vi "Module_p_control_v1.vi"() -> ()   [LabVIEW 2014]
uses:
  <vilib>/rvi/FXPMathLib/FxpSinAndCos/XNode/nifxpmath_SinAndCos.xnode
  <vilib>/eio/EIONode/EIONode.xnode
  <vilib>/rvi/FXPMathLib/FxpMul/XNode/nifxpmath_Multiplier.xnode
  <vilib>/rvi/FXPMathLib/FxpSinAndCos/simVIs/DllFxpSinAndCosTemp_sub.vi
  <vilib>/rvi/FXPMathLib/FxpSinAndCos/subVIs/nifxpmath_SinAndCos_SimConfig.ctl
  <vilib>/rvi/eio/common/nirviEmuTemplateMethod_errors.vi
  <vilib>/rvi/FXPMathLib/sim/FxpSim.dll
  <vilib>/rvi/DataTransferAndStorage/Container/XNode/niFpgaContainer.xnode
  <vilib>/rvi/FXPMathLib/FxpSub/XNode/nifxpmath_Sub.xnode
  <vilib>/rvi/FXPMathLib/FxpAdd/XNode/nifxpmath_Add.xnode
  <vilib>/rvi/Analysis/measure/butterworth/XNode/niFpgaButterworthFilter.xnode
  <vilib>/rvi/FXPMathLib/FxpAtan2/XNode/nifxpmath_Atan2.xnode
  <vilib>/rvi/FXPMathLib/FxpAtan2/simVIs/DllFxpAtan2Temp_sub.vi
  <vilib>/rvi/FXPMathLib/FxpAtan2/subVIs/nifxpmath_Atan2_SimConfig.ctl
  <vilib>/rvi/interface/RandomDataEmulation/nirviRandomDataFpgaMultiElementTemplate.vi
panel:
  out "Omega_p(M_avg)":fxp<+/-,57,22>
  out "Omega_p(M)":fxp<+/-,32,18>
  out "rad(NrTheta)_p":fxp<+/-,33,18>
  out "Encoder_Position_p":i32
  in  "fb_limit":fxp<+,16,11>
  in  "Dy_d_M_avg_Tc (uSec)":u32 caption="M_avg_Tc (uSec)"
  in  "Method case 2":i32
  out "Omega_b(rad/s)":fxp<+/-,32,18>
  out "Omega_y(M_avg)":fxp<+/-,32,18>
  out "Omega_y(M)":fxp<+/-,32,18>
  in  "Count(s)":u32
  out "Boolean":bool
  out "Db_temp":fxp<+/-,22,7>
  in  "Sin ini":bool
  out "xb_dd":fxp<+/-,25,15>
  in  "scaled coefficients_xb_dd":i32[](array[numeric])=[1067016412, 3362706]
  out "Db_dd":fxp<+/-,25,15>
  in  "scaled coefficients_Db_dd":i32[](array[numeric])=[1067016412, 3362706]
  out "Dab_edd":fxp<+/-,34,12>
  out "Dab_ed":fxp<+/-,33,10>
  out "fbr":fxp<+/-,20,10>
  in  "Kvb":fxp<+,15,8>
  in  "Bvb":fxp<+,15,8>
  out "Dab_e":fxp<+/-,26,11>
  in  "Dbr":fxp<+/-,22,8>
  in  "Inv./Pos.":bool
  out "Dabr_sin/cos":fxp<+/-,22,8>
  in  "Sin_offset_b":fxp<+/-,12,8>
  in  "Sin_magnitude_b":fxp<+/-,11,8>
  out "Dabr_d":fxp<+/-,33,10>
  out "Sin_omega":fxp<+,29,9>
  out "Dabr_dd":fxp<+/-,34,12>
  in  "Sin wave frenqueny (Hz)":fxp<+,21,5>
  out "Dy_d(M_avg method)":fxp<+/-,32,12>
  in  "Dy_d_M_Tc (mSec)":u32 format="%#_6f"
  out "Dy_d(M method)":fxp<+/-,32,12>
  out "Dp_d(M_avg method)":fxp<+/-,25,10>
  in  "Dp_d_M_avg_Tc (uSec)":u32 caption="M_avg_Tc (uSec)"
  out "Dp_d(M method)":fxp<+/-,25,10>
  in  "Dp_d_M_Tc (mSec)":u32 format="%#_6f"
  in  "Method case":i32
  out "xb_d(T method)":fxp<+/-,25,10>
  out "Dy_d(T method)":fxp<+/-,32,12>
  in  "mt0_velocity":u32
  out "mt_velocity":u32
  in  "mt0_omega":u32
  out "mt_omega":u32
  out "fbt_d":fxp<+/-,25,15>
  out "Db_d(mm/s)":fxp<+/-,32,12>
  out "xb_d(mm/s)":fxp<+/-,25,10>
  in  "dFb_PID_add":bool
  in  "scaled coefficients_dFb_PID":i32[](array[numeric])=[1067016412, 3362706]
  out "dFb_PID":fxp<+/-,25,15>
  out "Sin wave time (s)":fxp<+,64,32>
  in  "Encoder Reset_p":bool
  out "Dp(mm)":fxp<+/-,22,7>
  in  "Friction tolerance_b":fxp<+,12,4>
  in  "Coe Ini":bool
  in  "Encoder Reset_y":bool
  in  "Stop Motor_b":bool
  in  "viscous_cons_b":fxp<+/-,20,10>
  in  "fstb":fxp<+/-,15,6>
  in  "Db_d_tol":fxp<+,20,12>
  in  "Kib":fxp<+,27,10>
  in  "Kdb":fxp<+,26,2>
  in  "kb c":fxp<+,15,8>
  in  "kb t":fxp<+,15,8>
  out "fbt_i":fxp<+/-,34,18>
  in  "Kpb":fxp<+,11,7>=0.375
  in  "fv_coeff. b":fxp<+,13,1>
  out "Friction comp_b":fxp<+/-,20,10>
  in  "fcb":fxp<+/-,15,6>
  in  "fvb":fxp<+,20,12>
  out "kb":fxp<+,15,8>
  out "fb_tilde":fxp<+/-,21,11>
  out "Fb_PID":fxp<+/-,21,11>
  in  "fb_tolerance":fxp<+,32,9>=1.0
  out "Encoder Position_y":i32
  out "rad(NrTheta)_y":fxp<+/-,33,18> format="%.21g"
  out "Dy(mm)":fxp<+/-,22,7>
  out "Omega_y(T)":fxp<+/-,20,9>
  out "vq_b_F":fxp<+/-,20,5> format="%.57g"
  out "vd_b_F":fxp<+/-,20,5>
  out "va_b":fxp<+/-,20,5> format="%.21g"
  out "vb_b":fxp<+/-,20,5> format="%.21g"
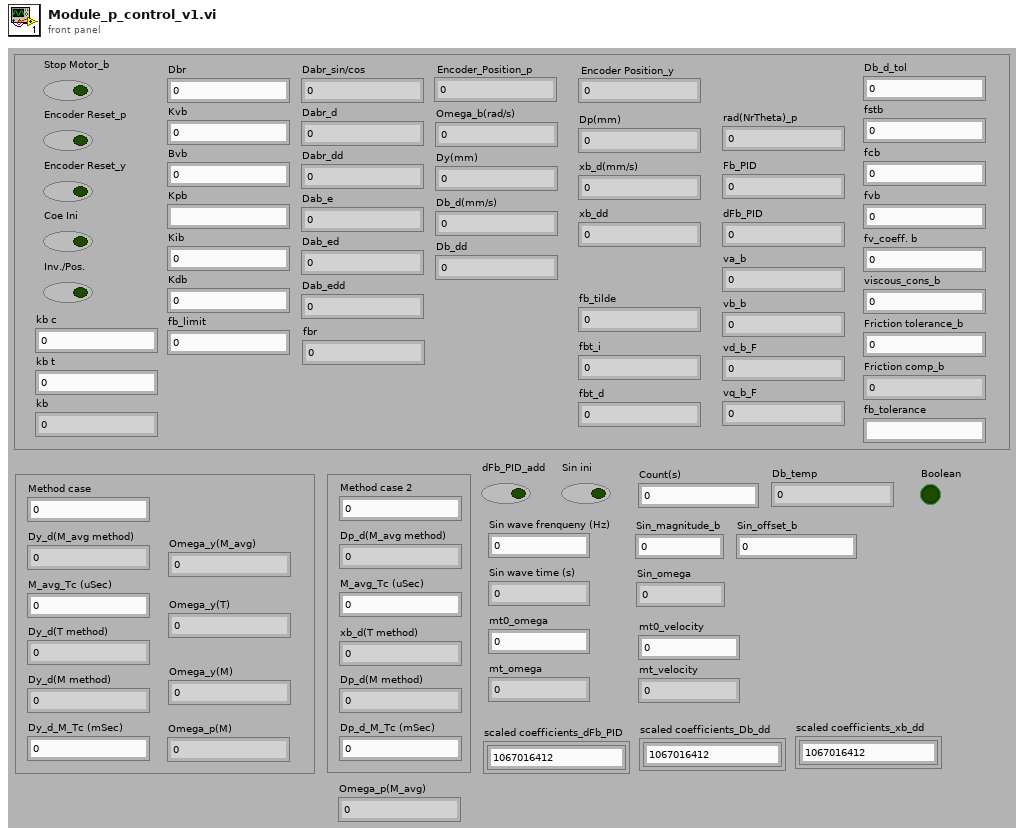
[diagram p1: front panel]
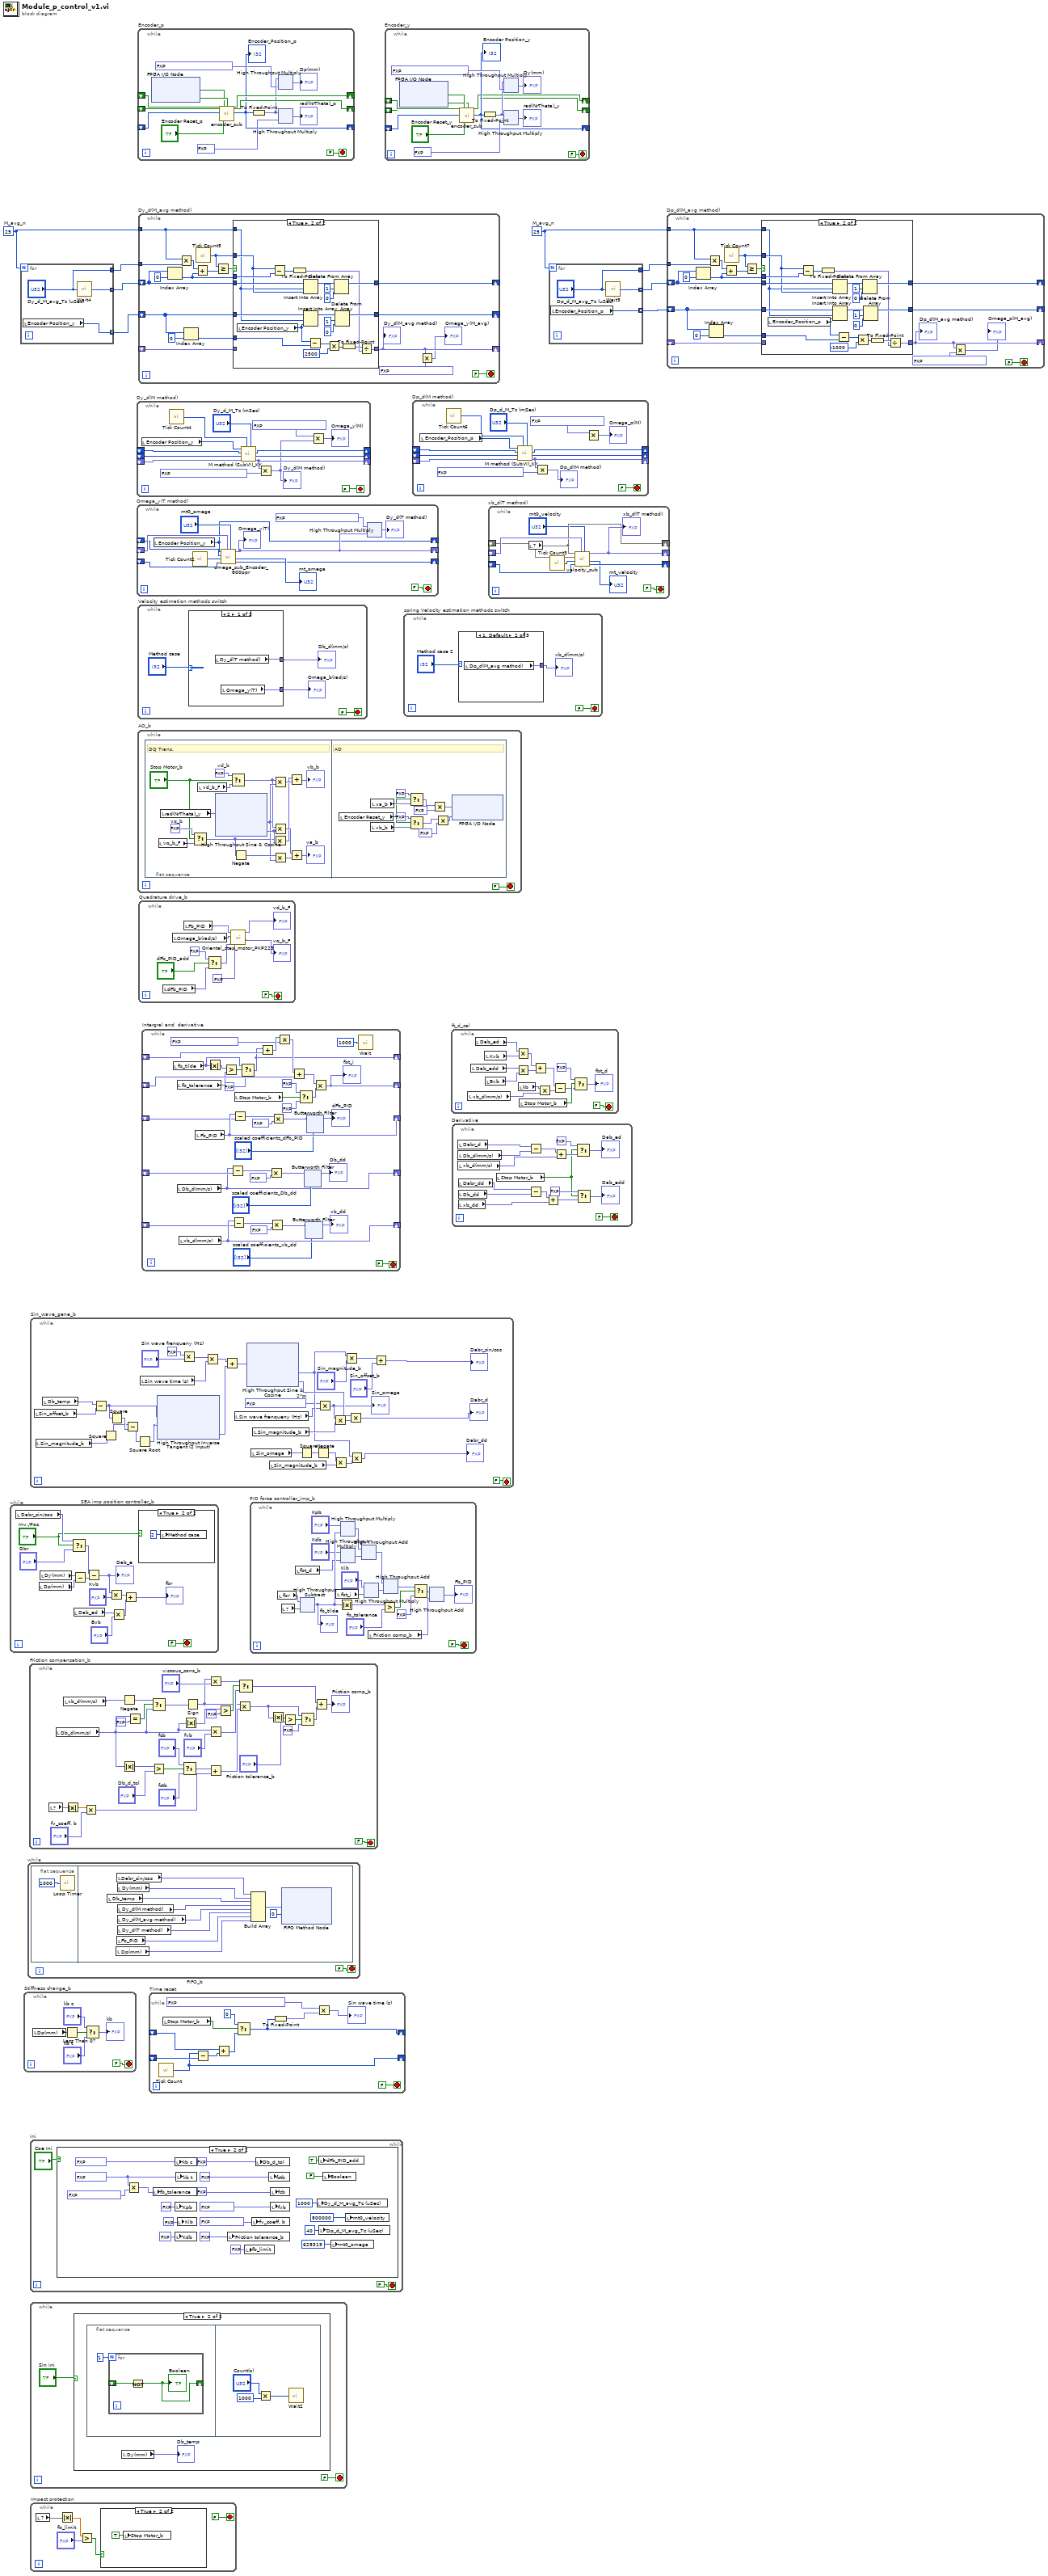
[diagram p0: block diagram]
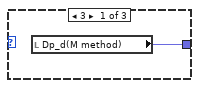
[diagram p4: hidden frame]
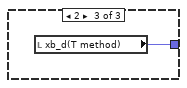
[diagram p5: hidden frame]
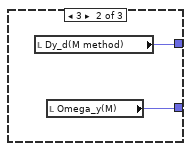
[diagram p9: hidden frame]
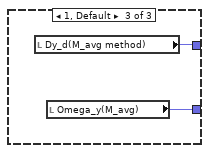
[diagram p10: hidden frame]
diagram:
  w3 = 25  # M_avg_n
  w7 = 25  # M_avg_n
  n1 = while "SEA imp position controller_b" {
    stop <- FALSE stop-if-true
    n2 = local read "Dabr_sin/cos"() -> (w11:fxp<+/-,22,8>)
    n3 = local read "Dp(mm)"() -> (w19:fxp<+/-,22,7>)
    n4 = local read "Dy(mm)"() -> (w18:fxp<+/-,22,7>)
    n5 = Select(t=w11, s="Inv./Pos.", f="Dbr") -> (s? t:f=w13:fxp<+/-,22,8>)
    n6 = Subtract(x=w18, y=w19) -> (x-y=w17:fxp<+/-,22,7>)
    n7 = local read "Dab_ed"() -> (w16:fxp<+/-,33,10>)
    n8 = Subtract(x=w13, y=w17) -> (x-y=w22:fxp<+/-,24,9>)
    "Dab_e" <- w22
    n9 = Multiply(x=w22, y="Kvb") -> (x*y=w20:fxp<+/-,39,17>)
    n10 = Multiply(x=w16, y="Bvb") -> (x*y=w21:fxp<+/-,48,18>)
    n11 = Add(x=w20, y=w21) -> (x+y=→"fbr":fxp<+/-,20,10>)
    n12 = case shown="True" "Inv./Pos." {
      frame False {
      }
      frame True {
        n13 = local write "Method case"(2 ("Method case")) -> ()
      }
    }
  }
  n14 = for {
    N: w3 -> [_]
    tunnel: [w27] -> w1 mode=indexing
    tunnel: [w25] -> w2 mode=indexing
    tunnel: ["Dy_d_M_avg_Tc (uSec)"] -> w4
    n15 = local read "Encoder Position_y"() -> (w25:i32)
    n16 = call "Wait4"("Count(uSec)"="Dy_d_M_avg_Tc (uSec)") -> ("Tick Count(uSec)"=w27:u32)
  }
  n17 = while "Stiffness change_b" {
    stop <- FALSE stop-if-true
    n18 = local read "Dp(mm)"() -> (w33:fxp<+/-,22,7>)
    n19 = Less Than 0?(x=w33) -> (x < 0?=w32:bool)
    n20 = Select(t="kb c", s=w32, f="kb t") -> (s? t:f=→"kb":fxp<+,15,8>)
  }
  n21 = while "FIFO_b" {
    stop <- FALSE stop-if-true
    n22 = flat-sequence {
      frame #0 {
        n23 = call "Loop Timer"("Count(uSec)"=u32 1000 ("Loop Period (usec)")) -> ()  [unwired: 1 out]
      }
      frame #1 {
        n24 = local read "Db_temp"() -> (w39:fxp<+/-,22,7>)
        n25 = local read "Dp(mm)"() -> (w44:fxp<+/-,22,7>)
        n26 = local read "Dabr_sin/cos"() -> (w41:fxp<+/-,22,8>)
        n27 = local read "Fb_PID"() -> (w37:fxp<+/-,21,11>)
        n28 = local read "Dy(mm)"() -> (w40:fxp<+/-,22,7>)
        n29 = local read "Dy_d(M method)"() -> (w45:fxp<+/-,32,12>)
        n30 = local read "Dy_d(M_avg method)"() -> (w38:fxp<+/-,32,12>)
        n31 = local read "Dy_d(T method)"() -> (w36:fxp<+/-,32,12>)
        n32 = Build Array(w41, w40, w39, w45, w38, w36, w37, w44) -> (w42:fxp<+/-,32,12>[])
        n33 = xnode ("FIFO Method Node")("Element"=w42, "Timeout"=0) -> ()  [unwired: 1 in, 2 out]
      }
    }
  }
  n34 = while "Friction compensation_b" {
    stop <- FALSE stop-if-true
    n35 = local read item#-1() -> (w75)
    n36 = local read "Db_d(mm/s)"() -> (w56:fxp<+/-,32,12>)
    n37 = local read "xb_d(mm/s)"() -> (w53:fxp<+/-,25,10>)
    n38 = Absolute Value(x=w75) -> (abs(x)=w76:dbl)
    n39 = Multiply(x=w76, y="fv_coeff. b") -> (x*y=w73:fxp<+/-,20,10>)
    n40 = Negate(x=w53) -> (-x=w52:fxp<+/-,26,11>)
    n41 = Absolute Value(x=w56) -> (abs(x)=w70:fxp<+,32,12>)
    n42 = Equal?(x=w56, y=fxp<+/-,25,15> 0.0) -> (x = y?=w57:bool)
    n43 = Select(t=w52, s=w57, f=w56) -> (s? t:f=w55:fxp<+/-,32,12>)
    n44 = Greater?(x=w70, y="Db_d_tol") -> (0:w69:bool)
    n45 = Select(t="fcb", s=w69, f="fstb") -> (s? t:f=w67:fxp<+/-,15,6>)
    n46 = Absolute Value(x=w56) -> (abs(x)=w64:fxp<+,32,12>)
    n47 = Sign(1:w55) -> (0:w54:fxp<+/-,2,2>)
    n48 = Multiply(x=w54, y="viscous_cons_b") -> (x*y=w59:fxp<+/-,20,10>)
    n49 = Multiply(x=w56, y="fvb") -> (x*y=w62:fxp<+/-,20,10>)
    n50 = Add(x=w67, y=w73) -> (x+y=w72:fxp<+/-,20,10>)
    n51 = Greater?(x=w64, y=fxp<+/-,25,15> 25.0) -> (0:w63:bool)
    n52 = Multiply(x=w54, y=w72) -> (x*y=w48:fxp<+/-,20,10>)
    n53 = Select(t=w59, s=w63, f=w62) -> (s? t:f=w61:fxp<+/-,20,10>)
    n54 = Absolute Value(x=w48) -> (abs(x)=w50:fxp<+,20,10>)
    n55 = Greater?(x=w50, y="Friction tolerance_b") -> (0:w51:bool)
    n56 = Select(t=w48, s=w51, f=fxp<+/-,20,10> 0.0) -> (s? t:f=w47:fxp<+/-,20,10>)
    n57 = Add(x=w61, y=w47) -> (x+y=→"Friction comp_b":fxp<+/-,20,10>)
  }
  n58 = while "ini" {
    stop <- FALSE stop-if-true
    n59 = case shown="True" "Coe Ini" {
      frame False {
      }
      frame True {
        w92 = fxp<+,15,8> 58.640625 ("kb")
        n60 = Multiply(x=w92, y=fxp<+,17,1> 0.00250244140625 ("kb")) -> (x*y=w93:fxp<+,32,9>)
        n61 = local write "fb_tolerance"(w93) -> ()
        n62 = local write "kb c"(fxp<+,15,8> 58.640625 ("kb")) -> ()
        n63 = local write "Kpb"(fxp<+,11,7> 40.0 ("Kpb")) -> ()
        n64 = local write "Kdb"(fxp<+,26,2> 0.5 ("Kdb")) -> ()
        n65 = local write "kb t"(w92) -> ()
        n66 = local write "Kib"(fxp<+,27,10> 20.0 ("Kib")) -> ()
        n67 = local write "Friction tolerance_b"(fxp<+,12,4> 10.0 ("Friction tolerance_y")) -> ()
        n68 = local write "fb_limit"(fxp<+,10,5> 10.0 ("fb_limit")) -> ()
        n69 = local write "fv_coeff. b"(fxp<+,13,1> 0.14990234375 ("fv_coeff. y")) -> ()
        n70 = local write "Db_d_tol"(fxp<+,20,12> 1.0 ("Dy_d_tol")) -> ()
        n71 = local write "fstb"(fxp<+/-,15,6> 12.0 ("fsty")) -> ()
        n72 = local write "fcb"(fxp<+/-,15,6> 8.0 ("fcy")) -> ()
        n73 = local write "fvb"(fxp<+,20,12> 0.19921875 ("fvy")) -> ()
        n74 = local write "Dy_d_M_avg_Tc (uSec)"(u32 1000 ("M_avg_Tc (uSec)")) -> ()
        n75 = local write "dFb_PID_add"(TRUE ("dF_PID_add")) -> ()
        n76 = local write "Dp_d_M_avg_Tc (uSec)"(u32 40 ("M_avg_Tc (uSec)")) -> ()
        n77 = local write "Boolean"(FALSE ("dF_PID_add")) -> ()
        n78 = local write "mt0_omega"(u32 628319 ("mt0_omega")) -> ()
        n79 = local write "mt0_velocity"(u32 800000 ("mt0_velocity")) -> ()
      }
    }
  }
  n80 = while {
    stop <- FALSE stop-if-true
    n81 = case shown="True" "Sin ini" {
      frame False {
      }
      frame True {
        n82 = flat-sequence {
          frame #0 {
            n83 = for {
              N: 1 -> [_]
              shift-right: [w106] -> _
              shift-left: _ -> [w107]
              n84 = Not(x=w107) -> (.not. x?=w106:bool)
              "Boolean" <- w106
            }
          }
          frame #1 {
            n85 = Multiply(x="Count(s)", y=u32 1000) -> (x*y=w108:u32)
            n86 = call "Wait2"("Count(mSec)"=w108) -> ()  [unwired: 1 out]
          }
        }
        n87 = local read "Dy(mm)"() -> (→"Db_temp":fxp<+/-,22,7>)
      }
    }
  }
  n88 = while "Sin_wave_gene_b" {
    stop <- FALSE stop-if-true
    w116 = fxp<+,20,3> 6.2831878662109375  # 2*pi
    n89 = local read "Sin_offset_b"() -> (w137:fxp<+/-,12,8>)
    n90 = local read "Sin_magnitude_b"() -> (w136:fxp<+/-,11,8>)
    n91 = local read "Db_temp"() -> (w138:fxp<+/-,22,7>)
    n92 = Subtract(x=w138, y=w137) -> (x-y=w135:fxp<+/-,24,9>)
    n93 = Square(x=w136) -> (x^2=w133:fxp<+,21,15>)
    n94 = Square(x=w135) -> (x^2=w134:fxp<+,46,16>)
    n95 = Subtract(x=w133, y=w134) -> (x-y=w132:fxp<+,47,17>)
    n96 = Square Root(x=w132) -> (sqrt(x)=w131:fxp<+,50,9>)
    n97 = local read "Sin wave time (s)"() -> (w118:fxp<+,64,32>)
    n98 = xnode "High Throughput Inverse Tangent (2 Input)"("y"=w135, "x"=w131) -> ("atan2(y,x) (pi)"=w139:fxp<+/-,16,2>)
    n99 = Multiply(x=fxp<+,1,2> 2.0 ("y"), y="Sin wave frenqueny (Hz)") -> (x*y=w119:fxp<+,21,6>)
    n100 = Multiply(x=w119, y=w118) -> (x*y=w117:fxp<+,48,18>)
    n101 = Add(x=w117, y=w139) -> (x+y=w140:fxp<+/-,50,20>)
    n102 = local read "Sin wave frenqueny (Hz)"() -> (w114:fxp<+,21,5>)
    n103 = xnode "High Throughput Sine & Cosine"("x (pi)"=w140) -> ("sin(x)"=w122:fxp<+/-,17,2>, "cos(x)"=w128:fxp<+/-,17,2>)
    n104 = local read "Sin_omega"() -> (w126:fxp<+,29,9>)
    n105 = local read "Sin_magnitude_b"() -> (w130:fxp<+/-,11,8>)
    n106 = local read "Sin_magnitude_b"() -> (w127:fxp<+/-,11,8>)
    n107 = Square(x=w126) -> (x^2=w125:fxp<+,35,15>)
    n108 = Negate(x=w125) -> (-x=w124:fxp<+/-,36,16>)
    n109 = Multiply(x=w116, y=w114) -> (x*y=w115:fxp<+,29,9>)
    "Sin_omega" <- w115
    n110 = Multiply(x=w115, y=w130) -> (x*y=w129:fxp<+,31,9>)
    n111 = Multiply(x=w124, y=w127) -> (x*y=w123:fxp<+/-,34,12>)
    n112 = Multiply(x=w122, y="Sin_magnitude_b") -> (x*y=w143:fxp<+/-,20,8>)
    n113 = Multiply(x=w128, y=w129) -> (x*y=→"Dabr_d":fxp<+/-,33,10>)
    n114 = Multiply(x=w122, y=w123) -> (x*y=→"Dabr_dd":fxp<+/-,34,12>)
    n115 = Add(x=w143, y="Sin_offset_b") -> (x+y=→"Dabr_sin/cos":fxp<+/-,22,8>)
  }
  n116 = while "Impact protection" {
    stop <- FALSE stop-if-true
    n117 = local read item#-1() -> (w206)
    n118 = Absolute Value(x=w206) -> (abs(x)=w205:dbl)
    n119 = Greater?(x=w205, y="fb_limit") -> (0:w203:bool)
    n120 = case shown="True" w203 {
      frame False {
      }
      frame True {
        n121 = local write "Stop Motor_b"(TRUE ("Stop Motor_b")) -> ()
      }
    }
  }
  n122 = while "Dy_d(M method)" {
    shift-right: [w220] -> _
    shift-left: _ -> [w215]
    shift-right: [w219] -> _
    shift-left: _ -> [w214]
    shift-right: [w212] -> _
    shift-left: _ -> [w213]
    stop <- FALSE stop-if-true
    n123 = local read "Encoder Position_y"() -> (w216:i32)
    n124 = call "Tick Count4"() -> ("Tick Count(mSec)"=w217:u32)
    n125 = call "M method (SubVI)_KY.vi"("Tc (mSec)"="Dy_d_M_Tc (mSec)", "Tick Count (mSec)"=w217, "Encoder velocity_pre (pulse/s)"=w213, "Shift Register in 2"=w214, "Shift Register in 1"=w215, "Encoder pulses"=w216) -> ("Encoder velocity (pulse/s)"=w212:fxp<+/-,64,32>, "Shift Register out 2"=w219:i32, "Shift Register out 1"=w220:u32)  [unwired: 3 in]
    n126 = Multiply(x=w212, y=fxp<+/-,20,-5> 0.002499997615814209) -> (x*y=w211:fxp<+/-,32,12>)
    "Dy_d(M method)" <- w211
    n127 = Multiply(x=fxp<+/-,32,12> 3.1415929794311523, y=w211) -> (x*y=→"Omega_y(M)":fxp<+/-,32,18>)
  }
  n128 = while "Omega_y(T method)" {
    shift-right: [w225] -> _
    shift-left: _ -> [w224]
    shift-right: [w223] -> _
    shift-left: _ -> [w230]
    shift-right: [w228] -> _
    shift-left: _ -> [w226]
    stop <- FALSE stop-if-true
    n129 = local read "Encoder Position_y"() -> (w225:i32)
    n130 = call "Tick Count2"() -> ("Tick Count(Ticks)"=w231:u32)
    n131 = call "omega_sub_Encoder_800ppr.vi"("mt0"="mt0_omega", "omega_pre"=w226, "ticks_m_pre"=w230, "ticks"=w231, "count_pre"=w224, "count"=w225) -> ("ticks_m"=w223:u32, "mt"=→"mt_omega":u32, "omega"=w228:fxp<+/-,20,9>)  [unwired: 3 in]
    "Omega_y(T)" <- w228
    n132 = xnode ("High Throughput Multiply")("x"=fxp<+/-,26,1> 0.3183099031448364, "y"=w228) -> ("x*y"=→"Dy_d(T method)":fxp<+/-,32,12>)
  }
  n133 = while "Encoder_p" {
    shift-right: [w245] -> _
    shift-left: _ -> [w246]
    shift-right: [w244] -> _
    shift-left: _ -> [w243]
    shift-right: [w240] -> _
    shift-left: _ -> [w241]
    stop <- FALSE stop-if-true
    n134 = xnode "FPGA I/O Node"() -> ("Mod4/DI0"=w247:bool, "Mod4/DI1"=w248:bool)  [unwired: 2 in, 2 out]
    n135 = call "encoder_sub.vi"("A_pre"=w246, "B_pre"=w243, "Encoder Position_pre"=w241, "A input"=w247, "Encoder Position Reset"="Encoder Reset_p", "B input"=w248) -> ("A"=w245:bool, "B"=w244:bool, "Encoder Position (Counts)"=w240:i32)  [unwired: 19 in]
    "Encoder_Position_p" <- w240
    n136 = To Fixed-Point(number=w240) -> (fixed-point=w238:fxp<+/-,32,32>)  [unwired: 1 in]
    n137 = xnode "High Throughput Multiply"("x"=w238, "y"=fxp<+/-,15,-7> 0.0025000572204589844) -> ("x*y"=→"Dp(mm)":fxp<+/-,33,18>)
    n138 = xnode "High Throughput Multiply"("x"=w238, "y"=fxp<+,16,1> 0.125) -> ("x*y"=→"rad(NrTheta)_p":fxp<+/-,33,18>)
  }
  n139 = while "Velocity estimation methods switch" {
    stop <- FALSE stop-if-true
    n140 = case shown="2" "Method case" {
      tunnel: [w254 w256 w258] -> w251
      tunnel: [w255 w257 w259] -> w250
      frame 2 {
        n141 = local read "Dy_d(T method)"() -> (w254:fxp<+/-,32,12>)
        n142 = local read "Omega_y(T)"() -> (w255:fxp<+/-,20,9>)
      }
      frame 3 {
        n143 = local read "Dy_d(M method)"() -> (w256:fxp<+/-,32,12>)
        n144 = local read "Omega_y(M)"() -> (w257:fxp<+/-,32,18>)
      }
      frame 1, Default {
        n145 = local read "Dy_d(M_avg method)"() -> (w258:fxp<+/-,32,12>)
        n146 = local read "Omega_y(M_avg)"() -> (w259:fxp<+/-,32,18>)
      }
    }
    "Db_d(mm/s)" <- w251
    "Omega_b(rad/s)" <- w250
  }
  n147 = while "AO_b" {
    stop <- FALSE stop-if-true
    n148 = flat-sequence {
      frame #0 {
        w267 = fxp<+/-,20,5> 0.0  # vq_b
        w266 = fxp<+/-,20,5> 0.0  # vd_b
        # "DQ Trans."
        n149 = local read "vq_b_F"() -> (w264:fxp<+/-,20,5>)
        n150 = local read "rad(NrTheta)_y"() -> (w277:fxp<+/-,33,18>)
        n151 = Select(t=w267, s="Stop Motor_b", f=w264) -> (s? t:f=w261:fxp<+/-,20,5>)
        n152 = local read "vd_b_F"() -> (w265:fxp<+/-,20,5>)
        n153 = xnode "High Throughput Sine & Cosine"("x (pi)"=w277) -> ("sin(x)"=w268:fxp<+/-,17,2>, "cos(x)"=w269:fxp<+/-,17,2>)
        n154 = Select(t=w266, s="Stop Motor_b", f=w265) -> (s? t:f=w262:fxp<+/-,20,5>)
        n155 = Negate(x=w261) -> (-x=w276:fxp<+/-,21,6>)
        n156 = Multiply(x=w262, y=w268) -> (x*y=w272:fxp<+/-,20,5>)
        n157 = Multiply(x=w262, y=w269) -> (x*y=w275:fxp<+/-,20,5>)
        n158 = Multiply(x=w261, y=w269) -> (x*y=w271:fxp<+/-,20,5>)
        n159 = Multiply(x=w276, y=w268) -> (x*y=w274:fxp<+/-,20,5>)
        n160 = Add(x=w271, y=w272) -> (x+y=→"vb_b":fxp<+/-,20,5>)
        n161 = Add(x=w275, y=w274) -> (x+y=→"va_b":fxp<+/-,20,5>)
      }
      frame #1 {
        # "AO"
        n162 = local read "Encoder Reset_y"() -> (w314:bool)
        n163 = local read "va_b"() -> (w315:fxp<+/-,20,5>)
        n164 = local read "vb_b"() -> (w316:fxp<+/-,20,5>)
        n165 = Select(t=fxp<+/-,20,5> 3.0 ("Mod2/AO4"), s=w314, f=w315) -> (s? t:f=w312:fxp<+/-,20,5>)
        n166 = Select(t=fxp<+/-,20,5> 0.0 ("Mod2/AO4"), s=w314, f=w316) -> (s? t:f=w309:fxp<+/-,20,5>)
        n167 = Multiply(x=w312, y=fxp<+/-,20,5> -0.5) -> (x*y=w313:fxp<+/-,20,5>)
        n168 = Multiply(x=w309, y=fxp<+/-,20,5> -0.5) -> (x*y=w308:fxp<+/-,20,5>)
        n169 = xnode "FPGA I/O Node"("Mod8/AO0"=w313, "Mod8/AO1"=w308) -> ()  [unwired: 2 in, 2 out]
      }
    }
  }
  n170 = while "Dy_d(M_avg method)" {
    shift-right: [w329] -> _
    shift-left: w1 -> [w332]
    tunnel: w3 -> [w330]
    shift-right: [w327] -> _
    shift-left: w2 -> [w325]
    shift-right: [w320] -> _
    shift-left: _ -> [w323]
    tunnel: w4 -> [w322]
    stop <- FALSE stop-if-true
    n171 = Index Array(array=w332, index=0) -> (element=w328:u32)
    n172 = Multiply(x=w330, y=w322) -> (x*y=w335:u32)
    n173 = Index Array(array=w325, index=0) -> (element=w324:i32)
    n174 = Add(x=w335, y=w328) -> (x+y=w334:u32)
    n175 = call "Tick Count5"() -> ("Tick Count(uSec)"=w331:u32)
    n176 = Greater Or Equal?(x=w331, y=w334) -> (x >= y?=w333:bool)
    n177 = case shown="True" w333 {
      tunnel: w332 -> [w340 w362]
      tunnel: w331 -> [_ w356]
      tunnel: w330 -> [_ w345]
      tunnel: [w340 w358] -> w329
      tunnel: w328 -> [_ w357]
      tunnel: w325 -> [w339 w346]
      tunnel: [w339 w344] -> w327
      tunnel: [w338 w343] -> w320
      tunnel: w324 -> [_ w341]
      tunnel: w323 -> [w338 _]
      frame False {
      }
      frame True {
        n178 = local read "Encoder Position_y"() -> (w350:i32)
        n179 = Subtract(x=w356, y=w357) -> (x-y=w355:u32)
        n180 = To Fixed-Point(number=w355) -> (fixed-point=w342:fxp<+,32,32>)  [unwired: 1 in]
        n181 = Insert Into Array(array=w362, index=w345, new element=w356) -> (w361:u32[])
        n182 = Insert Into Array(array=w346, index=w345, new element=w350) -> (w347:i32[])
        n183 = Subtract(x=w350, y=w341) -> (x-y=w351:i32)
        n184 = Multiply(x=w351, y=2500) -> (x*y=w353:i32)
        n185 = Delete From Array(array=w361, length=1, index=0) -> (array with subset deleted=w358:u32[])  [unwired: 1 out]
        n186 = Delete From Array(array=w347, length=1, index=0) -> (array with subset deleted=w344:i32[])  [unwired: 1 out]
        n187 = To Fixed-Point(number=w353) -> (fixed-point=w354:fxp<+/-,32,32>)  [unwired: 1 in]
        n188 = Divide(x=w354, y=w342) -> (x/y=w343:fxp<+/-,32,12>)
      }
    }
    "Dy_d(M_avg method)" <- w320
    n189 = Multiply(x=w320, y=fxp<+/-,32,12> 3.1415929794311523 ("x")) -> (x*y=→"Omega_y(M_avg)":fxp<+/-,32,18>)
  }
  n190 = while "Quadrature drive_b" {
    stop <- FALSE stop-if-true
    n191 = local read "dFb_PID"() -> (w369:fxp<+/-,25,15>)
    n192 = local read "Omega_b(rad/s)"() -> (w365:fxp<+/-,32,18>)
    n193 = local read "Fb_PID"() -> (w366:fxp<+/-,21,11>)
    n194 = Select(t=fxp<+/-,25,15> 0.0 ("f"), s="dFb_PID_add", f=w369) -> (s? t:f=w364:fxp<+/-,25,15>)
    n195 = call "Oriental_step_motor_PKP225.vi"("F_Threshold"=fxp<+,12,12> 10.0, "dFmr"=w364, "omega"=w365, "Fmr"=w366) -> ("vq_F"=→"vq_b_F":fxp<+/-,20,5>, "vd_F"=→"vd_b_F":fxp<+/-,20,5>)  [unwired: 6 in]
  }
  n196 = while "Intergral and  derivative" {
    shift-right: [w400] -> _
    shift-left: _ -> [w401]
    shift-right: [w387] -> _
    shift-left: _ -> [w406]
    shift-right: [w396] -> _
    shift-left: _ -> [w394]
    shift-right: [w380] -> _
    shift-left: _ -> [w381]
    shift-right: [w379] -> _
    shift-left: _ -> [w378]
    stop <- FALSE stop-if-true
    n197 = local read "fb_tilde"() -> (w402:fxp<+/-,21,11>)
    n198 = local read "fb_tolerance"() -> (w404:fxp<+,32,9>)
    n199 = local read "Db_d(mm/s)"() -> (w380:fxp<+/-,32,12>)
    n200 = local read "xb_d(mm/s)"() -> (w379:fxp<+/-,25,10>)
    n201 = local read "Fb_PID"() -> (w396:fxp<+/-,21,11>)
    n202 = Absolute Value(x=w402) -> (abs(x)=w405:fxp<+,21,11>)
    n203 = Greater?(x=w405, y=w404) -> (0:w403:bool)
    n204 = Subtract(x=w380, y=w381) -> (x-y=w383:fxp<+/-,33,13>)
    n205 = Subtract(x=w379, y=w378) -> (x-y=w376:fxp<+/-,26,11>)
    n206 = Subtract(x=w396, y=w394) -> (x-y=w395:fxp<+/-,22,12>)
    n207 = local read "Stop Motor_b"() -> (w408:bool)
    n208 = Select(t=w402, s=w403, f=fxp<+/-,21,11> 0.0) -> (s? t:f=w400:fxp<+/-,21,11>)
    n209 = Add(x=w400, y=w401) -> (x+y=w410:fxp<+/-,22,12>)
    n210 = Multiply(x=w383, y=fxp<+,10,10> 1000.0) -> (x*y=w384:fxp<+/-,25,15>)
    n211 = Multiply(x=w376, y=fxp<+,10,10> 1000.0) -> (x*y=w375:fxp<+/-,25,15>)
    n212 = Multiply(x=w395, y=fxp<+,10,10> 1000.0) -> (x*y=w393:fxp<+/-,25,15>)
    n213 = Multiply(x=w410, y=fxp<+/-,30,12> 0.000499725341796875) -> (x*y=w407:fxp<+/-,25,15>)
    n214 = Add(x=w407, y=w406) -> (x+y=w388:fxp<+/-,32,16>)
    n215 = Select(t=fxp<+/-,2,2> 0.0, s=w408, f=fxp<+/-,2,2> 1.0) -> (s? t:f=w389:fxp<+/-,2,2>)
    n216 = xnode "Butterworth Filter"("input data"=w384, "scaled coefficients"="scaled coefficients_Db_dd") -> ("output data"=→"Db_dd":fxp<+/-,25,15>)  [unwired: 1 in]
    n217 = xnode "Butterworth Filter"("input data"=w375, "scaled coefficients"="scaled coefficients_xb_dd") -> ("output data"=→"xb_dd":fxp<+/-,25,15>)  [unwired: 1 in]
    n218 = xnode "Butterworth Filter"("input data"=w393, "scaled coefficients"="scaled coefficients_dFb_PID") -> ("output data"=→"dFb_PID":fxp<+/-,25,15>)  [unwired: 1 in]
    n219 = Multiply(x=w388, y=w389) -> (x*y=w387:fxp<+/-,34,18>)
    "fbt_i" <- w387
    n220 = call "Wait"("Count(uSec)"=u32 1000 ("Count(mSec)")) -> ()  [unwired: 1 out]
  }
  n221 = while "Time reset" {
    shift-right: [w447] -> _
    shift-left: _ -> [w448]
    shift-right: [w439] -> _
    shift-left: _ -> [w441]
    stop <- FALSE stop-if-true
    n222 = call "Tick Count"() -> ("Tick Count(uSec)"=w447:u32)
    n223 = local read "Stop Motor_b"() -> (w444:bool)
    n224 = Subtract(x=w447, y=w448) -> (x-y=w443:u32)
    n225 = Add(x=w441, y=w443) -> (x+y=w442:u32)
    n226 = Select(t=u32 0, s=w444, f=w442) -> (s? t:f=w439:u32)
    n227 = To Fixed-Point(number=w439) -> (fixed-point=w437:fxp<+,64,32>)  [unwired: 1 in]
    n228 = Multiply(x=fxp<+,20,-18> 1.0000003385357559e-06 ("y"), y=w437) -> (x*y=→"Sin wave time (s)":fxp<+,64,32>)
  }
  n229 = while "PID force controller_imp_b" {
    stop <- FALSE stop-if-true
    n230 = local read "fbr"() -> (w452:fxp<+/-,20,10>)
    n231 = local read item#-1() -> (w463)
    n232 = local read "fbt_d"() -> (w450:fxp<+/-,25,15>)
    n233 = xnode "High Throughput Subtract"("x"=w452, "y"=w463) -> ("x-y"=w465:fxp<+/-,21,11>)
    "fb_tilde" <- w465
    n234 = local read "fbt_i"() -> (w461:fxp<+/-,34,18>)
    n235 = Absolute Value(x=w465) -> (abs(x)=w467:fxp<+,21,11>)
    n236 = xnode ("High Throughput Multiply")("x"="Kpb", "y"=w465) -> ("x*y"=w464:fxp<+/-,33,17>)
    n237 = xnode ("High Throughput Multiply")("x"="Kdb", "y"=w450) -> ("x*y"=w458:fxp<+/-,31,21>)
    n238 = xnode ("High Throughput Add")("x"=w464, "y"=w458) -> ("x+y"=w462:fxp<+/-,21,11>)
    n239 = xnode ("High Throughput Multiply")("x"="Kib", "y"=w461) -> ("x*y"=w460:fxp<+/-,31,14>)
    n240 = local read "Friction comp_b"() -> (w456:fxp<+/-,20,10>)
    n241 = Greater?(x=w467, y="fb_tolerance") -> (0:w466:bool)
    n242 = xnode ("High Throughput Add")("x"=w462, "y"=w460) -> ("x+y"=w459:fxp<+/-,21,11>)
    n243 = Select(t=w459, s=w466, f=fxp<+/-,21,11> 0.0) -> (s? t:f=w457:fxp<+/-,21,11>)
    n244 = xnode ("High Throughput Add")("x"=w457, "y"=w456) -> ("x+y"=→"Fb_PID":fxp<+/-,21,11>)
  }
  n245 = while "Encoder_y" {
    shift-right: [w471] -> _
    shift-left: _ -> [w483]
    shift-right: [w470] -> _
    shift-left: _ -> [w482]
    shift-right: [w475] -> _
    shift-left: _ -> [w481]
    stop <- FALSE stop-if-true
    n246 = xnode "FPGA I/O Node"() -> ("Mod4/DI2"=w473:bool, "Mod4/DI3"=w472:bool)  [unwired: 2 in, 2 out]
    n247 = call "encoder_sub.vi"("A_pre"=w483, "B_pre"=w482, "Encoder Position_pre"=w481, "A input"=w473, "Encoder Position Reset"="Encoder Reset_y", "B input"=w472) -> ("A"=w471:bool, "B"=w470:bool, "Encoder Position (Counts)"=w475:i32)  [unwired: 19 in]
    "Encoder Position_y" <- w475
    n248 = To Fixed-Point(number=w475) -> (fixed-point=w478:fxp<+/-,18,18>)  [unwired: 1 in]
    n249 = xnode ("High Throughput Multiply")("x"=w478, "y"=fxp<+/-,15,-7> 0.0025000572204589844) -> ("x*y"=→"Dy(mm)":fxp<+/-,22,7>)
    n250 = xnode ("High Throughput Multiply")("x"=w478, "y"=fxp<+,24,0> 0.125) -> ("x*y"=→"rad(NrTheta)_y":fxp<+/-,33,18>)
  }
  n251 = while "spring Velocity estimation methods switch" {
    stop <- FALSE stop-if-true
    n252 = case shown="1, Default" "Method case 2" {
      tunnel: [w488 w489 w490] -> w485
      frame 3 {
        n253 = local read "Dp_d(M method)"() -> (w488:fxp<+/-,25,10>)
      }
      frame 1, Default {
        n254 = local read "Dp_d(M_avg method)"() -> (w489:fxp<+/-,25,10>)
      }
      frame 2 {
        n255 = local read "xb_d(T method)"() -> (w490:fxp<+/-,25,10>)
      }
    }
    "xb_d(mm/s)" <- w485
  }
  n256 = while "Dp_d(M method)" {
    shift-right: [w501] -> _
    shift-left: _ -> [w496]
    shift-right: [w500] -> _
    shift-left: _ -> [w495]
    shift-right: [w493] -> _
    shift-left: _ -> [w494]
    stop <- FALSE stop-if-true
    n257 = local read "Encoder_Position_p"() -> (w497:i32)
    n258 = call "Tick Count6"() -> ("Tick Count(mSec)"=w498:u32)
    n259 = call "M method (SubVI)_KY.vi"("Tc (mSec)"="Dp_d_M_Tc (mSec)", "Tick Count (mSec)"=w498, "Encoder velocity_pre (pulse/s)"=w494, "Shift Register in 2"=w495, "Shift Register in 1"=w496, "Encoder pulses"=w497) -> ("Encoder velocity (pulse/s)"=w493:fxp<+/-,64,32>, "Shift Register out 2"=w500:i32, "Shift Register out 1"=w501:u32)  [unwired: 3 in]
    n260 = Multiply(x=w493, y=fxp<+/-,20,-5> 0.002499997615814209) -> (x*y=→"Dp_d(M method)":fxp<+/-,25,10>)
    n261 = Multiply(x=fxp<+,22,2> 3.1415929794311523) -> (x*y=→"Omega_p(M)":fxp<+,44,4>)  [unwired: 1 in]
  }
  n262 = while "ft_d_cal" {
    stop <- FALSE stop-if-true
    n263 = local read "xb_d(mm/s)"() -> (w517:fxp<+/-,25,10>)
    n264 = local read "Dab_edd"() -> (w511:fxp<+/-,34,12>)
    n265 = local read "Dab_ed"() -> (w512:fxp<+/-,33,10>)
    n266 = local read "Kvb"() -> (w510:fxp<+,15,8>)
    n267 = local read "Bvb"() -> (w509:fxp<+,15,8>)
    n268 = Multiply(x=w512, y=w510) -> (x*y=w514:fxp<+/-,48,18>)
    n269 = Multiply(x=w511, y=w509) -> (x*y=w515:fxp<+/-,49,20>)
    n270 = local read "kb"() -> (w518:fxp<+,15,8>)
    n271 = local read "Stop Motor_b"() -> (w508:bool)
    n272 = Add(x=w514, y=w515) -> (x+y=w516:fxp<+/-,51,21>)
    n273 = Multiply(x=w518, y=w517) -> (x*y=w519:fxp<+/-,35,12>)
    n274 = Subtract(x=w516, y=w519) -> (x-y=w507:fxp<+/-,25,15>)
    n275 = Select(t=fxp<+/-,25,15> 0.0, s=w508, f=w507) -> (s? t:f=→"fbt_d":fxp<+/-,25,15>)
  }
  n276 = while "Derivative" {
    stop <- FALSE stop-if-true
    n277 = local read "Dabr_d"() -> (w532:fxp<+/-,33,10>)
    n278 = local read "Db_d(mm/s)"() -> (w533:fxp<+/-,32,12>)
    n279 = local read "xb_d(mm/s)"() -> (w535:fxp<+/-,25,10>)
    n280 = local read "Dabr_dd"() -> (w530:fxp<+/-,34,12>)
    n281 = local read "Db_dd"() -> (w529:fxp<+/-,25,15>)
    n282 = local read "xb_dd"() -> (w527:fxp<+/-,25,15>)
    n283 = local read "Stop Motor_b"() -> (w520:bool)
    n284 = Subtract(x=w532, y=w533) -> (x-y=w534:fxp<+/-,33,10>)
    n285 = Subtract(x=w530, y=w529) -> (x-y=w528:fxp<+/-,38,16>)
    n286 = Add(x=w528, y=w527) -> (x+y=w524:fxp<+/-,34,12>)
    n287 = Add(x=w534, y=w535) -> (x+y=w526:fxp<+/-,33,10>)
    n288 = Select(t=fxp<+/-,33,10> 0.0, s=w520, f=w526) -> (s? t:f=→"Dab_ed":fxp<+/-,33,10>)
    n289 = Select(t=fxp<+/-,34,12> 0.0, s=w520, f=w524) -> (s? t:f=→"Dab_edd":fxp<+/-,34,12>)
  }
  n290 = while "xb_d(T method)" {
    shift-right: [w541] -> _
    shift-left: _ -> [w540]
    shift-right: [w543] -> _
    shift-left: _ -> [w538]
    shift-right: [w544] -> _
    shift-left: _ -> [w542]
    stop <- FALSE stop-if-true
    n291 = local read item#-1() -> (w541)
    n292 = call "Tick Count3"() -> ("Tick Count(Ticks)"=w539:u32)
    n293 = call "velocity_sub.vi"("mt0"="mt0_velocity", "velocity_pre"=w542, "ticks_m_pre"=w538, "ticks"=w539, "count_pre"=w540, "count"=w541) -> ("ticks_m"=w543:u32, "mt"=→"mt_velocity":u32, "velocity (mm/s)"=w544:fxp<+/-,25,10>)  [unwired: 3 in]
    "xb_d(T method)" <- w544
  }
  n294 = for {
    N: w7 -> [_]
    tunnel: [w548] -> w8 mode=indexing
    tunnel: ["Dp_d_M_avg_Tc (uSec)"] -> w6
    tunnel: [w546] -> w5 mode=indexing
    n295 = local read "Encoder_Position_p"() -> (w546:i32)
    n296 = call "Wait3"("Count(uSec)"="Dp_d_M_avg_Tc (uSec)") -> ("Tick Count(uSec)"=w548:u32)
  }
  n297 = while "Dp_d(M_avg method)" {
    shift-right: [w558] -> _
    shift-left: w8 -> [w561]
    shift-right: [w553] -> _
    shift-left: w5 -> [w555]
    tunnel: w7 -> [w559]
    shift-right: [w551] -> _
    shift-left: _ -> [w554]
    tunnel: w6 -> [w552]
    stop <- FALSE stop-if-true
    n298 = Index Array(array=w561, index=0) -> (element=w557:u32)
    n299 = Multiply(x=w559, y=w552) -> (x*y=w564:u32)
    n300 = Index Array(array=w555, index=0) -> (element=w556:i32)
    n301 = Add(x=w564, y=w557) -> (x+y=w563:u32)
    n302 = call "Tick Count7"() -> ("Tick Count(uSec)"=w560:u32)
    n303 = Greater Or Equal?(x=w560, y=w563) -> (x >= y?=w562:bool)
    n304 = case shown="True" w562 {
      tunnel: w561 -> [w570 w592]
      tunnel: w560 -> [_ w586]
      tunnel: w559 -> [_ w572]
      tunnel: [w570 w588] -> w558
      tunnel: w557 -> [_ w587]
      tunnel: w555 -> [w569 w583]
      tunnel: w556 -> [_ w579]
      tunnel: [w568 w574] -> w551
      tunnel: w554 -> [w568 _]
      tunnel: [w569 w573] -> w553
      frame False {
      }
      frame True {
        n305 = local read "Encoder_Position_p"() -> (w580:i32)
        n306 = Subtract(x=w586, y=w587) -> (x-y=w585:u32)
        n307 = To Fixed-Point(number=w585) -> (fixed-point=w571:fxp<+,32,32>)  [unwired: 1 in]
        n308 = Insert Into Array(array=w592, index=w572, new element=w586) -> (w591:u32[])
        n309 = Insert Into Array(array=w583, index=w572, new element=w580) -> (w584:i32[])
        n310 = Subtract(x=w580, y=w579) -> (x-y=w578:i32)
        n311 = Multiply(x=w578, y=-1000) -> (x*y=w576:i32)
        n312 = Delete From Array(array=w591, length=1, index=0) -> (array with subset deleted=w588:u32[])  [unwired: 1 out]
        n313 = Delete From Array(array=w584, length=1, index=0) -> (array with subset deleted=w573:i32[])  [unwired: 1 out]
        n314 = To Fixed-Point(number=w576) -> (fixed-point=w575:fxp<+/-,32,32>)  [unwired: 1 in]
        n315 = Divide(x=w575, y=w571) -> (x/y=w574:fxp<+/-,25,10>)
      }
    }
    "Dp_d(M_avg method)" <- w551
    n316 = Multiply(x=w551, y=fxp<+/-,32,12> 3.1415929794311523) -> (x*y=→"Omega_p(M_avg)":fxp<+/-,57,22>)
  }
